vi "Extract Lines.vi"(7 "Extraction mode":i32(knob) scale=0.0..2.0, 8 "error in (no error)":errorcluster, 11 "Image Src":T1) -> (0 "error out":errorcluster, 2 "Number of Particles1":i32, 3 "Image Out":T1)   [LabVIEW 2009]
doc: "VI which takes an image and outputs marked regions. One for the left and one for the right"
uses:
  <vilib>/vision/Image Controls.llb/IMAQ Image.ctl
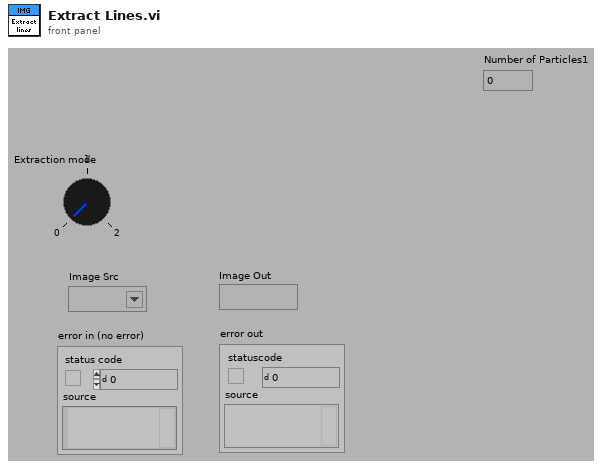
[diagram p1: front panel]
types:
  T1 = typedef "IMAQ Image.ctl" = refnum<image>
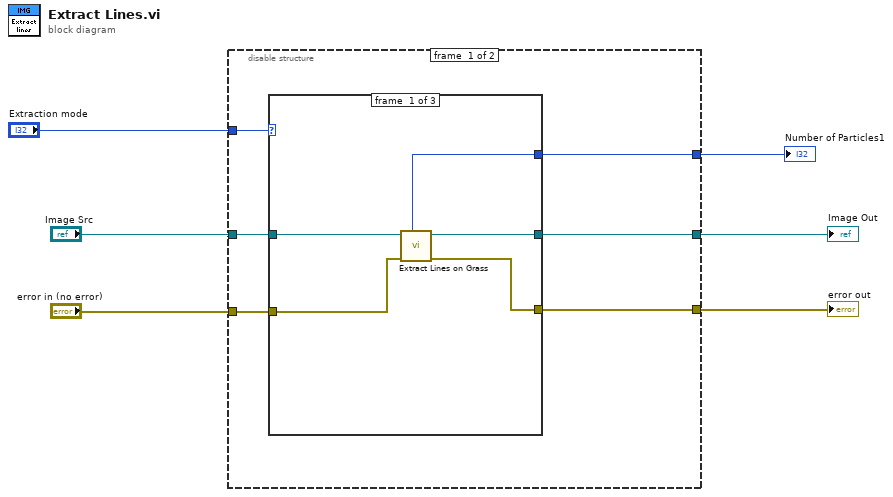
[diagram p0: block diagram]
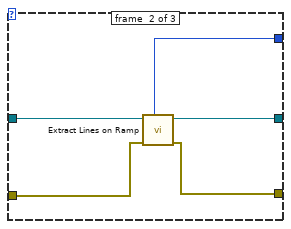
[diagram p2: hidden frame]
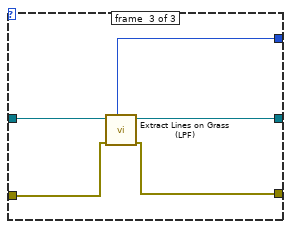
[diagram p3: hidden frame]
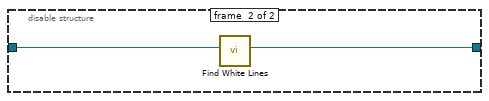
[diagram p4: hidden frame]
diagram:
  n1 = disable-structure shown="Enabled" {
    disable-tunnel: "Image Src" -> [w12 w29]
    disable-tunnel: "error in (no error)" -> [w11 _]
    disable-tunnel: [w10 _] -> w4
    disable-tunnel: [w9 _] -> w3
    disable-tunnel: "Extraction mode" -> [w8 _]
    disable-tunnel: [w7 w28] -> w1
    frame #0 {
      n2 = case shown="2" w8 {
        tunnel: w12 -> [w17 w22 w27]
        tunnel: w11 -> [w16 w21 w26]
        tunnel: [w15 w19 w25] -> w7
        tunnel: [w14 w20 w24] -> w10
        tunnel: [w13 w18 w23] -> w9
        frame #0 {
          n3 = call "Extract Lines on Grass.vi"("error in (no error)"=w16, "Image Src"=w17) -> ("error out"=w14:errorcluster, "Image Out"=w15:T1, "Number of Particles1"=w13:i32)  [unwired: 6 in, 1 out]
        }
        frame #1 {
          n4 = call "Extract Lines on Ramp.vi"("error in"=w21, "Image In"=w22) -> ("error out"=w20:errorcluster, "Image Out"=w19:T1, "Number of Particles"=w18:i32)  [unwired: 5 in]
        }
        frame #2 {
          n5 = call "Extract Lines on Grass (LPF).vi"("error in"=w26, "Image In"=w27) -> ("error out"=w24:errorcluster, "Image Out"=w25:T1, "Number of Particles"=w23:i32)  [unwired: 5 in]
        }
      }
    }
    frame #1 {
      n6 = call "Find White Lines.vi"("Image Src"=w29) -> ("Image"=w28:T1)  [unwired: 10 in]
    }
  }
  "error out" <- w4
  "Number of Particles1" <- w3
  "Image Out" <- w1
